vi "Parse Path Object Items.vi"(9 "error in (no error)":errorcluster, 11 "Path with leading Object element":string) -> (1 "error out":errorcluster, 2 "<JSON>items names":string[](array[string]), 3 "Rest or Path":string)   [LabVIEW 2017, in "JSONtext.lvlib"]
uses:
  JSONtext.lvlib
  Parsing State.ctl
  support/quote and escape json string 2.vi
  <vilib>/JDP Science/JDP Science Common Utilities/JDP Utility.lvlib
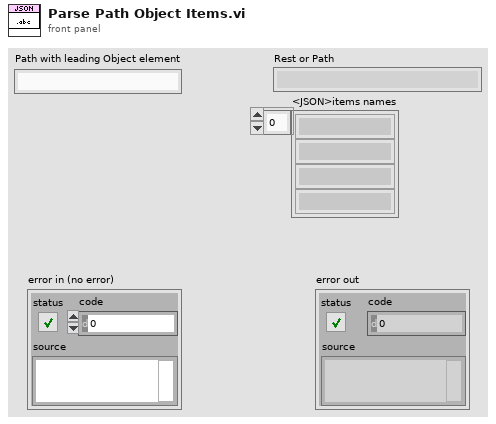
[diagram p1: front panel]
types:
  T1 = typedef "JSONtext.lvlib/Parsing State.ctl" = enum16{"Parser Error", "Object", "Array", "String", "Number/Other", "Leading Whitespace", "Object end", "Array end", "Value end"}
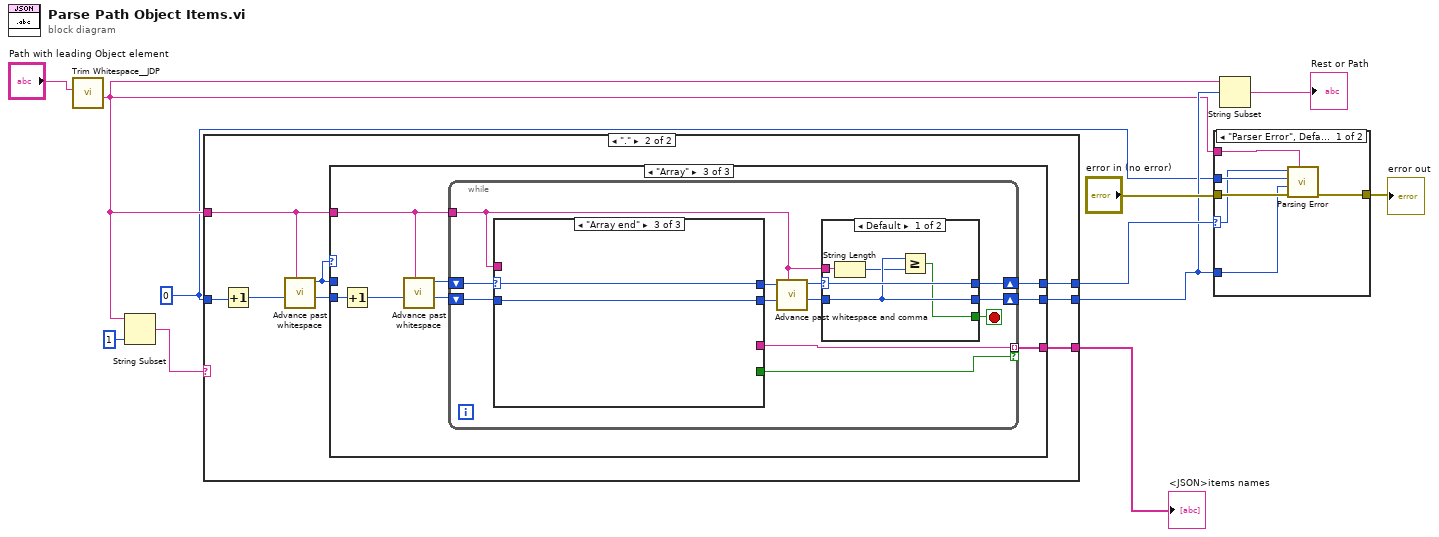
[diagram p0: block diagram]
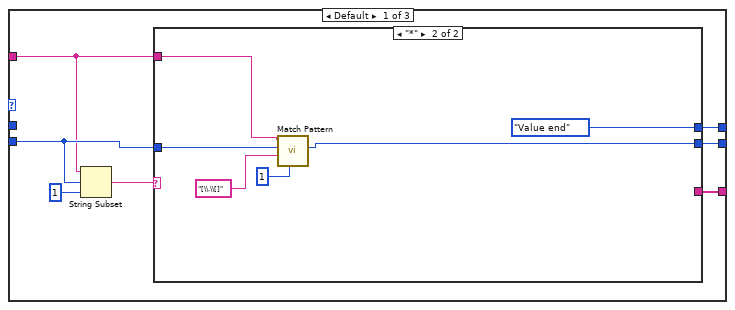
[diagram p4: hidden frame]
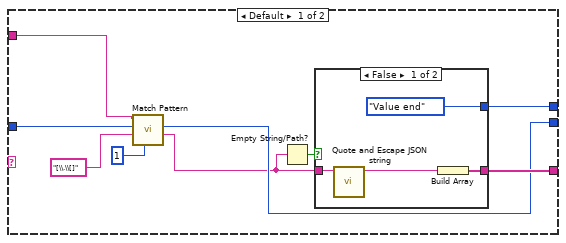
[diagram p5: hidden frame]
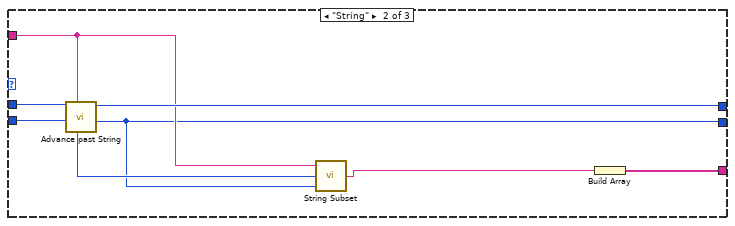
[diagram p7: hidden frame]
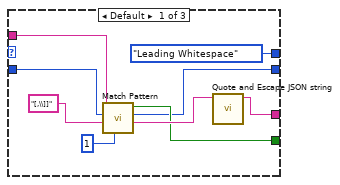
[diagram p8: hidden frame]
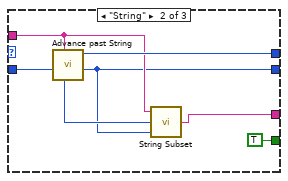
[diagram p9: hidden frame]
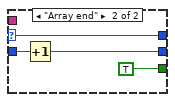
[diagram p10: hidden frame]
diagram:
  w2 = 0
  n1 = call <vilib>:"Trim Whitespace__JDP.vi"("String in"="Path with leading Object element") -> ("String out"=w4:string)  [unwired: 6 in]
  n2 = String Subset(string=w4, length (rest)=1 ("length (rest)")) -> (substring=w1:string)  [unwired: 1 in]
  n3 = case shown="\".\"" w1 {
    tunnel: w2 -> [w12 w20]
    tunnel: w4 -> [_ w18]
    tunnel: [_ w17] -> w8
    tunnel: [w12 w16] -> w7
    tunnel: [_ w13] -> w9
    frame Default {
    }
    frame "." {
      n4 = Increment(x=w20) -> (x+1=w19:i32)
      n5 = call "Advance past whitespace.vi"("JSON"=w18, "Offset"=w19) -> ("Offset of first non-whitespace"=w15:i32, "Parser State"=w14:T1)  [unwired: 8 in]
      n6 = case shown="\"Array\"" w14 {
        tunnel: w14 -> [_ w54 _]
        tunnel: w18 -> [w22 w51 w55]
        tunnel: w15 -> [w23 w53 w62]
        tunnel: [w27 w47 w61] -> w17
        tunnel: [w26 w49 w60] -> w16
        tunnel: [w25 w52 w59] -> w13
        frame Default {
          n7 = String Subset(string=w22, offset (0)=w23, length (rest)=1 ("length (rest)")) -> (substring=w21:string)
          n8 = case shown="\"*\"" w21 {
            tunnel: [w36 _] -> w27
            tunnel: [w34 w45] -> w26
            tunnel: [w33 Parsing_State."Value end" ("Parser State")] -> w25
            tunnel: w23 -> [w29 w42]
            tunnel: w22 -> [w28 w41]
            frame Default {
              n9 = call "Match Pattern.vi"("trim back if found"=1, "regular expression"="[\\.\\[]", "Offset in"=w29, "String in"=w28) -> ("substring"=w31:string, "Offset of match"=w34:i32)  [unwired: 5 in, 1 out]
              n10 = Empty String/Path?(string/path=w31) -> (empty?=w32:bool)
              n11 = case shown="False" w32 {
                tunnel: [w39 _] -> w36
                tunnel: w31 -> [w38 _]
                tunnel: [Parsing_State."Value end" ("Parser State") _] -> w33
                frame False {
                  n12 = call "Quote and Escape JSON string.vi"("Plain Text"=w38) -> ("<JSON>"=w40:string)  [unwired: 10 in]
                  n13 = Build Array(w40) -> (w39:string[])
                }
                frame True {
                }
              }
            }
            frame "*" {
              n14 = call "Match Pattern.vi"("trim back if found"=1, "regular expression"="[\\.\\[]", "Offset in"=w42, "String in"=w41) -> ("Offset of match"=w45:i32)  [unwired: 5 in, 2 out]
            }
          }
        }
        frame "String" {
          n15 = call "Advance past String.vi"("JSON"=w51, "Offset"=w53, "State in"=w54) -> ("Offset past match"=w49:i32, "State"=w52:T1, "Value start out"=w50:i32)  [unwired: 6 in]
          n16 = call "String Subset.vi"("Offset past End"=w49, "Start offset"=w50, "JSON"=w51) -> ("substring"=w48:string)  [unwired: 2 in]
          n17 = Build Array(w48) -> (w47:string[])
        }
        frame "Array" {
          n18 = Increment(x=w62) -> (x+1=w56:i32)
          n19 = call "Advance past whitespace.vi"("JSON"=w55, "Offset"=w56) -> ("Offset of first non-whitespace"=w57:i32, "Parser State"=w58:T1)  [unwired: 8 in]
          n20 = while {
            tunnel: w55 -> [w63]
            shift-right: [w72] -> w60
            shift-left: w57 -> [w66]
            shift-right: [w68] -> w59
            shift-left: w58 -> [w67]
            tunnel: [w65] -> w61 mode=indexing if=w64
            stop <- w71 stop-if-true
            n21 = case shown="\"Array end\"" w67 {
              selector: w67 -> [_ _ w92]
              tunnel: w66 -> [w80 w89 w91]
              tunnel: [Parsing_State."Leading Whitespace" ("State") w90 w92] -> w70
              tunnel: [w75 w86 w91] -> w69
              tunnel: w63 -> [w82 w88 _]
              tunnel: [w81 w85 _] -> w65
              tunnel: [w78 TRUE ("Found") _] -> w64
              frame Default {
                n22 = call "Match Pattern.vi"("trim back if found"=1, "regular expression"="[,\\]]", "Offset in"=w80, "String in"=w82) -> ("substring"=w79:string, "Offset of match"=w75:i32, "Found"=w78:bool)  [unwired: 5 in]
                n23 = call "Quote and Escape JSON string.vi"("Plain Text"=w79) -> ("<JSON>"=w81:string)  [unwired: 10 in]
              }
              frame "String" {
                n24 = call "Advance past String.vi"("JSON"=w88, "Offset"=w89) -> ("Offset past match"=w86:i32, "State"=w90:T1, "Value start out"=w87:i32)  [unwired: 7 in]
                n25 = call "String Subset.vi"("Offset past End"=w86, "Start offset"=w87, "JSON"=w88) -> ("substring"=w85:string)  [unwired: 2 in]
              }
              frame "Array end" {
              }
            }
            n26 = call "Advance past whitespace and comma.vi"("JSON"=w63, "Offset"=w69, "State in"=w70) -> ("Offset past match"=w74:i32, "State"=w73:T1)  [unwired: 7 in]
            n27 = case shown="Default" w73 {
              selector: w73 -> [w97 w98]
              tunnel: [w93 TRUE] -> w71
              tunnel: w74 -> [w96 w100]
              tunnel: [w96 w99] -> w72
              tunnel: [w97 w98] -> w68
              tunnel: w63 -> [w94 _]
              frame Default {
                n28 = String Length(string=w94) -> (length=w95:i32)
                n29 = Greater Or Equal?(x=w96, y=w95) -> (x >= y?=w93:bool)
              }
              frame "Array end" {
                n30 = Increment(x=w100) -> (x+1=w99:i32)
              }
            }
          }
        }
      }
    }
  }
  "<JSON>items names" <- w8
  n31 = case shown="\"Parser Error\", Default" w9 {
    selector: w9 -> [w102 _]
    tunnel: w4 -> [w107 _]
    tunnel: "error in (no error)" -> [w106 w108]
    tunnel: [w105 w108] -> w10
    tunnel: w2 -> [w104 _]
    tunnel: w7 -> [w103 _]
    frame "Parser Error", Default {
      n32 = call "Parsing Error.vi"("JSON"=w107, "error in (no error)"=w106, "Offset past match"=w103, "Value start"=w104, "State"=w102) -> ("error out"=w105:errorcluster)  [unwired: 6 in]
    }
    frame "Array end", "Value end" {
    }
  }
  "error out" <- w10
  n33 = String Subset(string=w4, offset (0)=w7) -> (substring=→"Rest or Path":string)  [unwired: 1 in]
